vi "Set Keys.vi"(8 "error in":errorcluster, 10 "Keys":refnum<class "Key Name.lvclass">[](array[class]), 11 "Object Entry in":refnum<class "Section.lvclass">) -> (0 "error out":errorcluster, 3 "Object Entry out":refnum<class "Section.lvclass">)   [LabVIEW 2024, in "Electronic Datasheet.lvlib" / "Section.lvclass"]
uses:
  Section.lvclass
  Keyname/Key Name.lvclass
  Section.lvclass/Section.ctl
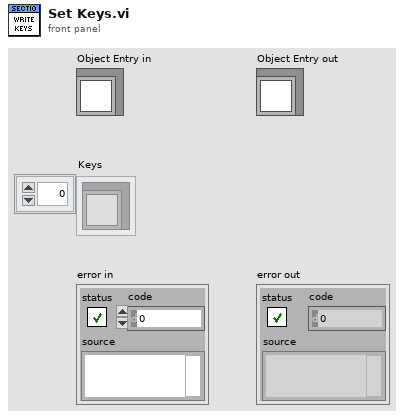
[diagram p1: front panel]
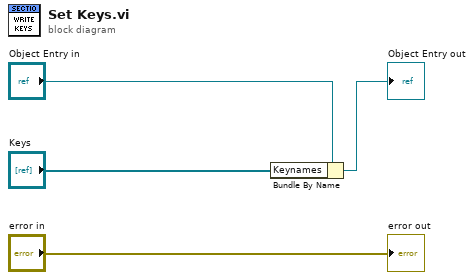
[diagram p0: block diagram]
diagram:
  n1 = Bundle By Name(cluster="Object Entry in", "Keynames"="Keys") -> (→"Object Entry out":refnum<class "Section.lvclass">)
  "error out" <- "error in"
